vi "RT_Boolean_Changed.vi"(11 "Boolean in":bool) -> (0 "Value":bool, 3 "Changed?":bool)   [LabVIEW 2020]
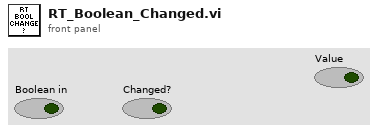
[diagram p1: front panel]
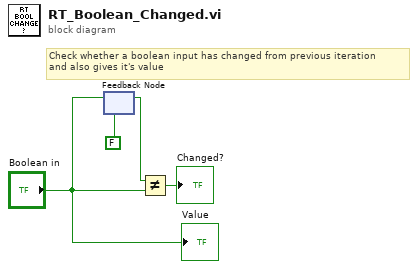
[diagram p0: block diagram]
diagram:
  # "Check whether a boolean input has changed from previous iteration\nand also gives it's value"
  n1 = feedback #1(FALSE ("Boolean")) -> (w1:bool)
  n2 = feedback-in #1("Boolean in") -> ()
  n3 = Not Equal?(x=w1, y="Boolean in") -> (x != y?=→"Changed?":bool)
  "Value" <- "Boolean in"
